vi "FTW-Test-CSV-ArrayOfClusters.vi"() -> ()   [LabVIEW 2015]
panel:
  out "CSV String":string
  out "error out":errorcluster
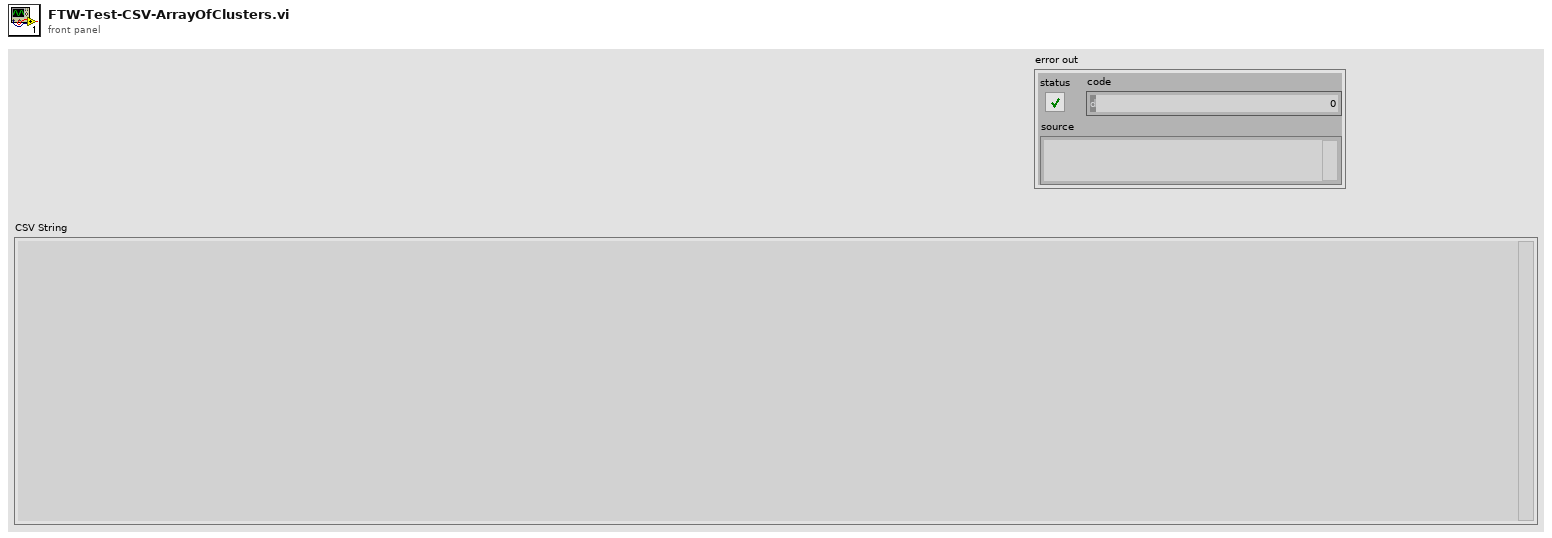
[diagram p1: front panel]
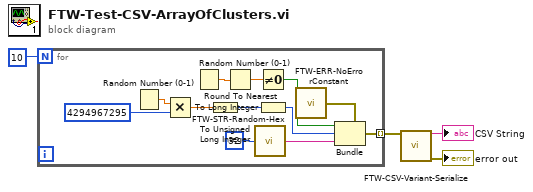
[diagram p0: block diagram]
diagram:
  n1 = for {
    N: 10 -> [_]
    tunnel: [w12] -> w1 mode=indexing
    n2 = Random Number (0-1)() -> (number: 0 to 1=w16:dbl)
    n3 = Multiply(x=w16, y=u32 4294967295) -> (x*y=w14:dbl)
    n4 = Random Number (0-1)() -> (number: 0 to 1=w10:dbl)
    n5 = To Unsigned Long Integer(number=w14) -> (unsigned 32bit integer=w5:u32)
    n6 = Round To Nearest(number=w10) -> (nearest integer value=w9:dbl)
    n7 = call "FTW-STR-Random-Hex.vi"("String Length"=32) -> ("Random Hex String"=w11:string)  [unwired: 3 in]
    n8 = Not Equal To 0?(x=w9) -> (x != 0?=w8:bool)
    n9 = To Long Integer(number=w5) -> (32bit integer=w13:i32)
    n10 = call "FTW-ERR-NoErrorConstant.vi"() -> ("no error"=w7:errorcluster)
    n11 = Bundle(cluster=w7, "status"=w8, "code"=w13, "source"=w11) -> (w12:errorcluster)
  }
  n12 = call "FTW-CSV-Variant-Serialize.vi"("Variant"=w1) -> ("CSV String"=→"CSV String":string, "error out"=→"error out":errorcluster)  [unwired: 13 in]
